vi "Wait.vi"(2 "Wartezeit in ms":u32, 3 "error in (no error)":errorcluster, 4 "Skip on Error":bool) -> (0 "error out":errorcluster)   [LabVIEW 2017]
doc: "This VI waits the specified time (in ms) (\"Pause\")"
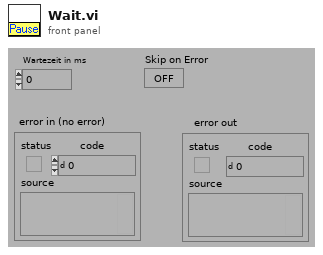
[diagram p1: front panel]
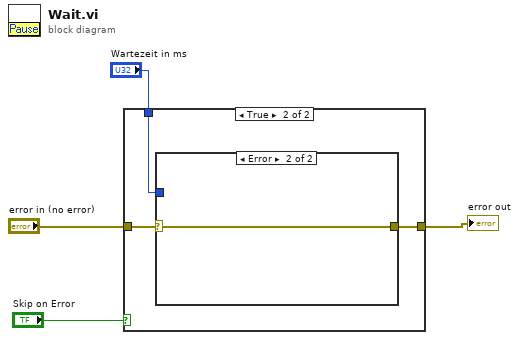
[diagram p0: block diagram]
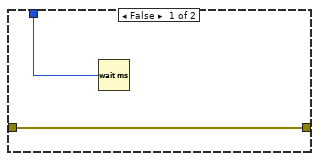
[diagram p2: hidden frame]
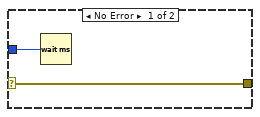
[diagram p3: hidden frame]
diagram:
  n1 = case shown="True" "Skip on Error" {
    tunnel: "error in (no error)" -> [w5 w9]
    tunnel: [w5 w8] -> w2
    tunnel: "Wartezeit in ms" -> [w6 w7]
    frame False {
      n2 = Wait (ms)(milliseconds to wait=w6) -> ()  [unwired: 1 out]
    }
    frame True {
      n3 = case shown="Error" w9 {
        selector: w9 -> [w11 w12]
        tunnel: [w11 w12] -> w8
        tunnel: w7 -> [w10 _]
        frame No Error {
          n4 = Wait (ms)(milliseconds to wait=w10) -> ()  [unwired: 1 out]
        }
        frame Error {
        }
      }
    }
  }
  "error out" <- w2
